vi "Init.vi"(8 "error in":errorcluster, 11 "NEOXID480HTA in":refnum<class "NEOXID480.lvclass">) -> (0 "error out":errorcluster, 3 "NEOXID480HTA out":refnum<class "NEOXID480.lvclass">)   [LabVIEW 2024, in "NEOXID480.lvclass"]
uses:
  NEOXID480.lvclass
  NEOXID480.lvclass/NEOXID480.ctl
  Source/Interfaces/IInstrument/IInstrument.lvclass
  Source/Instrument Factory/Instrument Factory.lvclass
  Source/DBCCommunication/DBC Communication.lvclass
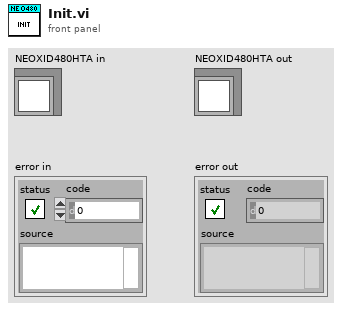
[diagram p1: front panel]
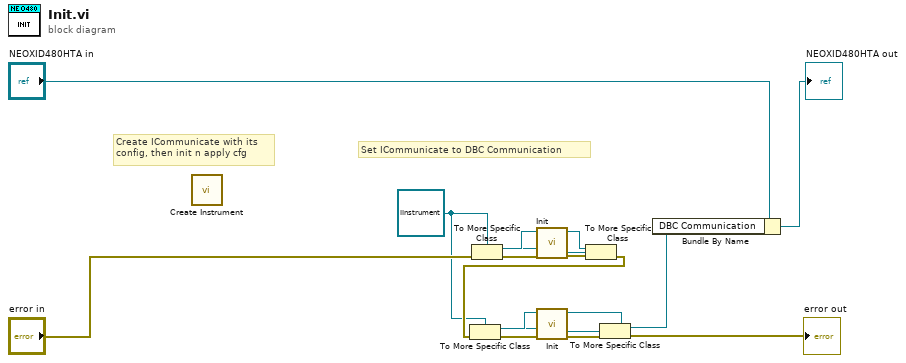
[diagram p0: block diagram]
diagram:
  w8 = refnum<class "IInstrument.lvclass"> refnum ("IInstrument.lvclass")
  # "Set ICommunicate to DBC Communication"
  # "Create ICommunicate with its\nconfig, then init n apply cfg"
  n1 = call "Create Instrument.vi"() -> ()  [unwired: 8 in, 4 out]
  n2 = To More Specific Class(target class=w8, error in=w9) -> (reference=w2:refnum<vi>, specific class reference=w7:refnum<class "IInstrument.lvclass">, error out=w15:errorcluster)
  n3 = call-dynamic "Init.vi"("error in"=w15, "IInstrument in"=w7) -> ("error out"=w6:errorcluster, "IInstrument out"=w3:refnum<class "IInstrument.lvclass">)  [unwired: 8 in]
  n4 = To More Specific Class(target class=w2, reference=w3, error in=w6) -> (specific class reference=w1:refnum<vi>, error out=→"error out":errorcluster)
  n5 = Bundle By Name(cluster="NEOXID480HTA in", "DBC Communication"=w1) -> (→"NEOXID480HTA out":refnum<class "NEOXID480.lvclass">)
  n6 = To More Specific Class(target class=w8, reference=w4, error in="error in") -> (specific class reference=w14:refnum<class "IInstrument.lvclass">, error out=w13:errorcluster)
  n7 = call-dynamic "Init.vi"("error in"=w13, "IInstrument in"=w14) -> ("error out"=w11:errorcluster, "IInstrument out"=w12:refnum<class "IInstrument.lvclass">)  [unwired: 8 in]
  n8 = To More Specific Class(reference=w12, error in=w11) -> (target class=w4:refnum<vi>, error out=w9:errorcluster)  [unwired: 1 out]
